vi "Encoder.vi"() -> ()   [LabVIEW 2017]
uses:
  <vilib>/DAQmx/read.llb/DAQmx Read (Counter DBL 1Chan 1Samp).vi
  <vilib>/DAQmx/create/channels.llb/DAQmx Create Channel (CI-Count Edges).vi
  <vilib>/DAQmx/miscellaneous.llb/DAQmx Fill In Error Info.vi
panel:
  out "data":dbl format="%0.2f"
  in  "stop":bool
  out "error out":errorcluster
  in  "error in (no error)":errorcluster
  in  "Test":bool
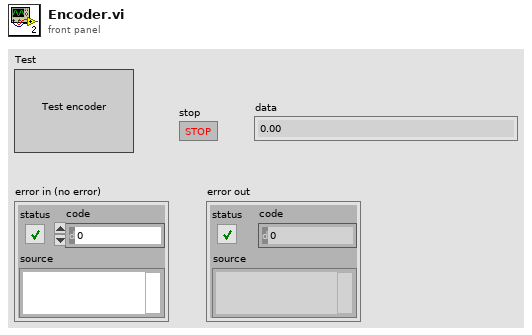
[diagram p1: front panel]
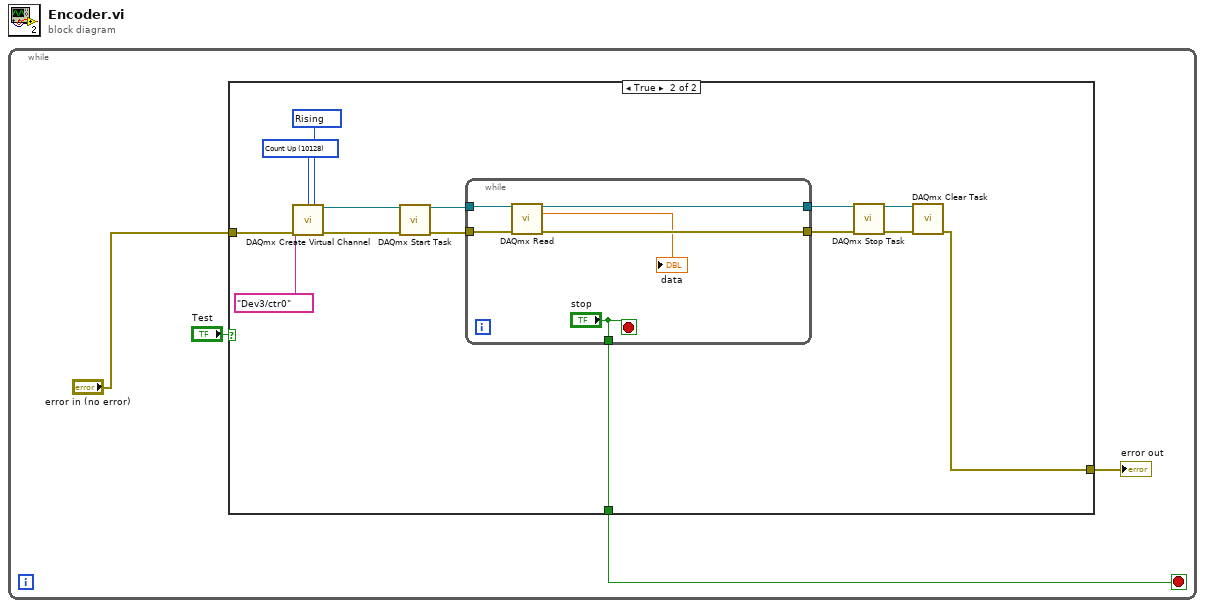
[diagram p0: block diagram]
diagram:
  n1 = while {
    stop <- w1 stop-if-true
    n2 = case shown="True" "Test" {
      tunnel: "error in (no error)" -> [_ w14]
      tunnel: [_ w9] -> w2
      tunnel: [_ w8] -> w1
      frame False {
      }
      frame True {
        w7 = 10128 items=["Count Up"=10128, "Count Down"=10124, "Externally Controlled"=10326] ("count direction")
        w6 = 10280 items=["Rising"=10280, "Falling"=10171] ("edge")
        n3 = call-poly <vilib>:"DAQmx Create Virtual Channel.vi"("count direction"=w7, "edge"=w6, "counter"=tag "Dev3/ctr0", "error in"=w14) -> ("task out"=w5:refnum<k21>, "error out"=w16:errorcluster)  [unwired: 10 in]
        n4 = call <vilib>:"DAQmx Start Task.vi"("task/channels in"=w5, "error in"=w16) -> ("task out"=w18:refnum<k21>, "error out"=w17:errorcluster)  [unwired: 12 in]
        n5 = while {
          tunnel: w17 -> [w23]
          tunnel: [w21] -> w12
          tunnel: w18 -> [w24]
          tunnel: [w22] -> w13
          tunnel: ["stop"] -> w8
          stop <- "stop" stop-if-true
          n6 = call-poly <vilib>:"DAQmx Read.vi"("task/channels in"=w24, "error in"=w23) -> ("task out"=w22:refnum<k21>, "data"=→"data":dbl, "error out"=w21:errorcluster)  [unwired: 11 in]
        }
        n7 = call <vilib>:"DAQmx Stop Task.vi"("task/channels in"=w13, "error in"=w12) -> ("task out"=w11:refnum<k21>, "error out"=w10:errorcluster)  [unwired: 12 in]
        n8 = call <vilib>:"DAQmx Clear Task.vi"("task in"=w11, "error in"=w10) -> ("error out"=w9:errorcluster)  [unwired: 13 in]
      }
    }
    "error out" <- w2
  }
